vi "Replace Row In File.vi"(10 "Insert Array":dbl[][](array[numeric]), 11 "Path":path) -> (0 "error out":errorcluster)   [LabVIEW 2016]
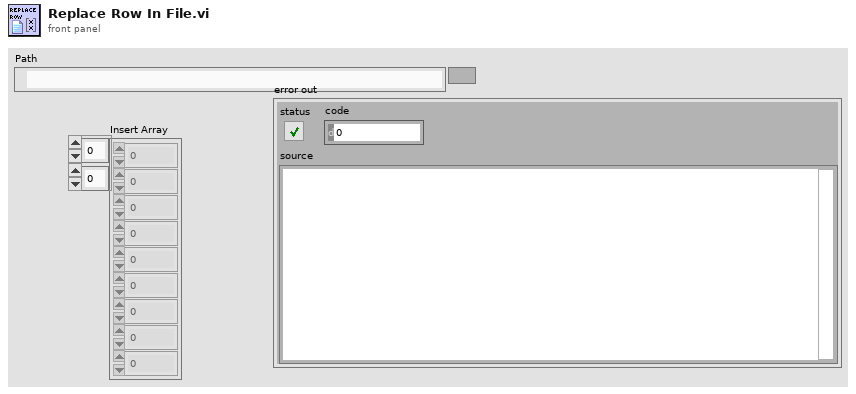
[diagram p1: front panel]
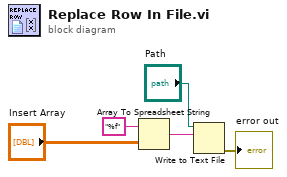
[diagram p0: block diagram]
diagram:
  n1 = Array To Spreadsheet String(array="Insert Array", 3:"%f" ("format string")) -> (spreadsheet string=w5:string)  [unwired: 1 in]
  n2 = Write to Text File(file (use dialog)="Path", text=w5) -> (error out=→"error out":errorcluster)  [unwired: 2 in, 2 out]
